vi "430_TCP_Query.vi"(8 "error in (no error)":errorcluster, 9 "Timeout":i32=1000, 10 "Command":string, 11 "connection ID":refnum<k5>) -> (0 "error out":errorcluster, 1 "Bytes Read":i32, 2 "Response":string, 3 "connection ID out":refnum<k5>, 4 "Bytes Written":i32)   [LabVIEW 2011]
panel:
  in  "error out 3":errorcluster
  out "error out 2":errorcluster
  out "data out":string
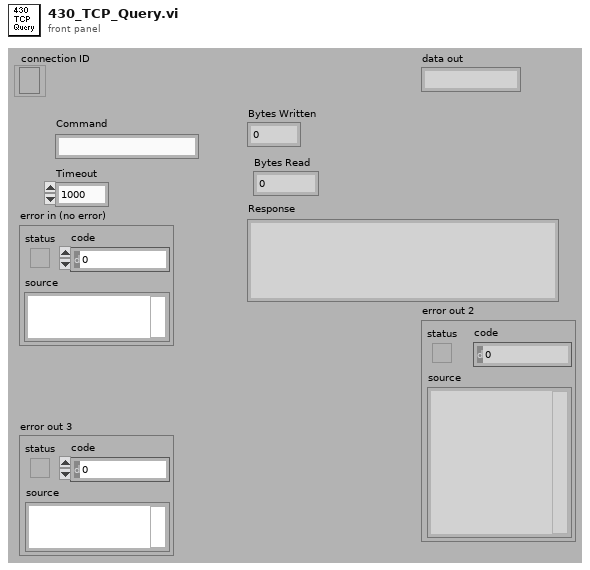
[diagram p1: front panel]
types:
  T1 = enum16{"Standard", "Buffered", "CRLF", "Immediate"}
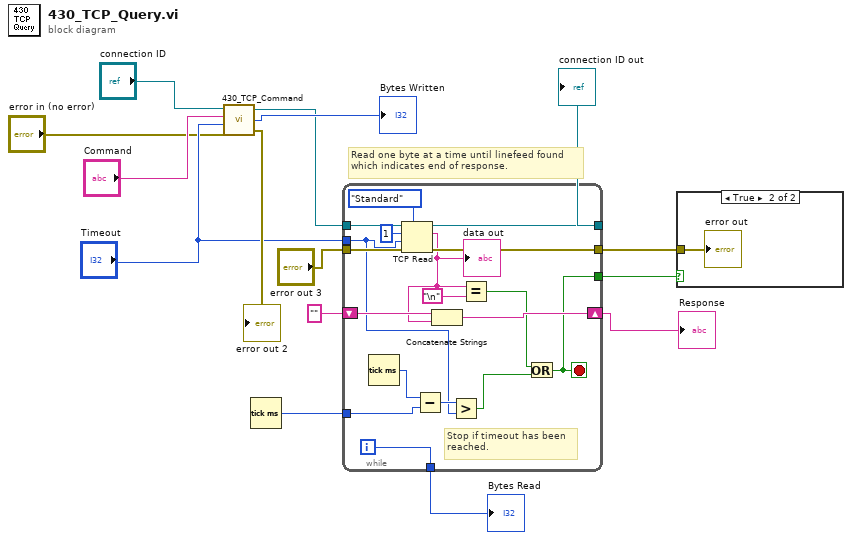
[diagram p0: block diagram]
diagram:
  # "Read one byte at a time until linefeed found\nwhich indicates end of response."
  n1 = call "430_TCP_Command.vi"("error in (no error)"="error in (no error)", "Timeout"="Timeout", "Command"="Command", "connection ID"="connection ID") -> ("error out"=→"error out 2":errorcluster, "bytes written"=→"Bytes Written":i32, "connection ID out"=w13:refnum<k5>)
  n2 = Tick Count (ms)() -> (millisecond timer value=w6:u32)
  n3 = while {
    tunnel: w13 -> [w33]
    tunnel: [w32] -> w12
    tunnel: "error out 3" -> [w31]
    tunnel: [w30] -> w10
    tunnel: [w29] -> w9
    shift-right: [w23] -> w7
    shift-left: "" -> [w25]
    tunnel: "Timeout" -> [w18]
    tunnel: w6 -> [w21]
    tunnel: [w17] -> w5
    i -> [w29]
    stop <- w17 stop-if-true
    # "Stop if timeout has been\nreached."
    n4 = Tick Count (ms)() -> (millisecond timer value=w22:u32)
    n5 = TCP Read(connection ID=w33, bytes to read=1, error in (no error)=w31, 7:T1."Standard" ("mode (standard)"), 9:w18) -> (connection ID out=w32:refnum<k5>, data out=w24:string, error out=w30:errorcluster)
    "data out" <- w24
    n6 = Subtract(x=w22, y=w21) -> (x-y=w20:u32)
    n7 = Concatenate Strings(w25, w24) -> (w23:string)
    n8 = Greater?(x=w20, y=w18) -> (0:w19:bool)
    n9 = Equal?(x=w24, y="\n") -> (x = y?=w16:bool)
    n10 = Or(x=w16, y=w19) -> (x .or. y?=w17:bool)
  }
  "Bytes Read" <- w9
  "Response" <- w7
  "connection ID out" <- w12
  n11 = case shown="True" w5 {
    tunnel: w10 -> [_ w34]
    frame False {
    }
    frame True {
      "error out" <- w34
    }
  }
